vi "Read Counter Input PWM Module.vi"(8 "error in":errorcluster, 11 "module in":refnum<class "Module.lvclass">) -> (0 "error out":errorcluster, 2 "channel settings":T1[](array[typedef]), 3 "module out":refnum<class "Module.lvclass">)   [LabVIEW 2020, in "Scan Engine Scripting.lvlib" / "Module.lvclass"]
uses:
  Module.lvclass
  Mode Classes/Controls/counter input pwm channel settings.ctl
  Channel Classes/PWM Input Channel/Measurement Type.ctl
  Mode Classes/Counter Input PWM Mode/Counter Input PWM Mode.lvclass
  Channel Classes/PWM Input Channel/PWM Input Channel.lvclass
  Scan Engine Scripting.lvlib
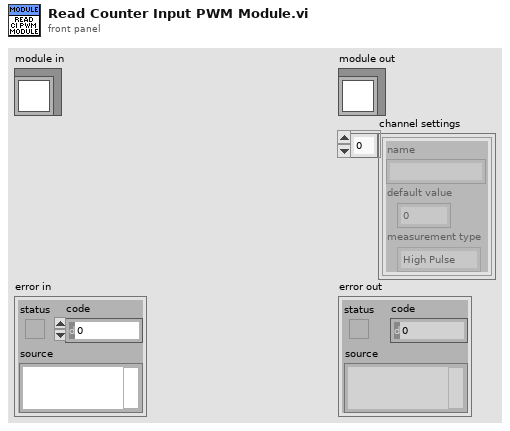
[diagram p1: front panel]
types:
  T1 = typedef "Scan Engine Scripting.lvlib/counter input pwm channel settings.ctl" = cluster{"name":string, "default value":dbl, "measurement type":T2}
  T2 = typedef "Scan Engine Scripting.lvlib/PWM Input Channel.lvclass/Measurement Type.ctl" = enum16{"High Pulse", "Low Pulse", "Most Recent"}
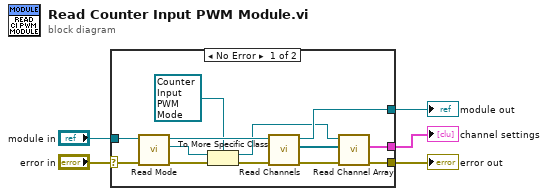
[diagram p0: block diagram]
diagram:
  n1 = case shown="No Error" "error in" {
    selector: "error in" -> [w17 w20]
    tunnel: [w9 w20] -> w2
    tunnel: [w13 w19] -> w3
    tunnel: "module in" -> [w18 w19]
    tunnel: [w6 _] -> w1
    frame No Error {
      n2 = call-dynamic "Read Mode.vi"("error in"=w17, "module in"=w18) -> ("error out"=w15:errorcluster, "mode"=w16:refnum<class "Mode.lvclass">, "module out"=w14:refnum<class "Module.lvclass">)  [unwired: 7 in]
      n3 = To More Specific Class(target class=refnum<class "Counter Input PWM Mode.lvclass"> refnum ("Scan Engine Scripting.lvlib:Analog Input Vrms Mode.lvclass"), reference=w16, error in=w15) -> (specific class reference=w7:refnum<class "Counter Input PWM Mode.lvclass">, error out=w10:errorcluster)
      n4 = call-dynamic "Read Channels.vi"("error in"=w10, "module in"=w14) -> ("error out"=w11:errorcluster, "channels"=w8:refnum<class "Channel.lvclass">[], "module out"=w13:refnum<class "Module.lvclass">)  [unwired: 7 in]
      n5 = call "Read Channel Array.vi"("error in"=w11, "channels"=w8, "counter input PWM mode in"=w7) -> ("error out"=w9:errorcluster, "channel settings"=w6:T1[])  [unwired: 6 in, 1 out]
    }
    frame Error {
    }
  }
  "error out" <- w2
  "module out" <- w3
  "channel settings" <- w1
